vi "MH_T2 Read Acq Q_V2.vi"() -> ()   [LabVIEW 2019]
uses:
  <userlib>/MultiHarp150/T2Lib/MH_T2DeltaQMessage.ctl
  <userlib>/MultiHarp150/T2Lib/MH_T2QMessage.ctl
  <userlib>/MultiHarp150/T2Lib/MH_ResizeBuffer.vi
panel:
  in  "buffbits":i32=16
  out "SpBufSze":i32=1000000
  in  "Dbuffsize":i32=100000
  out "Done":bool
  out "TotalRec":i32
  out "TotalTime":u32
  in  "stop":bool
  out "sortie d'erreur":errorcluster caption="ErrorOut"
  out "RollOver":bool
  out "StBufSze":i32=1000000
  in  "entrée d'erreur":errorcluster caption="ErrorIn"
  in  "WIndowW":i32
  in  "Save Data":bool
  in  "StopCh":u32=2
  in  "StartCh":u32=1
  in  "refnum":refnum<file>
  out "DeltaT":u32[](array[numeric])
  out "nActual":i32[](array[numeric])
  out "En Attente":i32[](array[numeric])
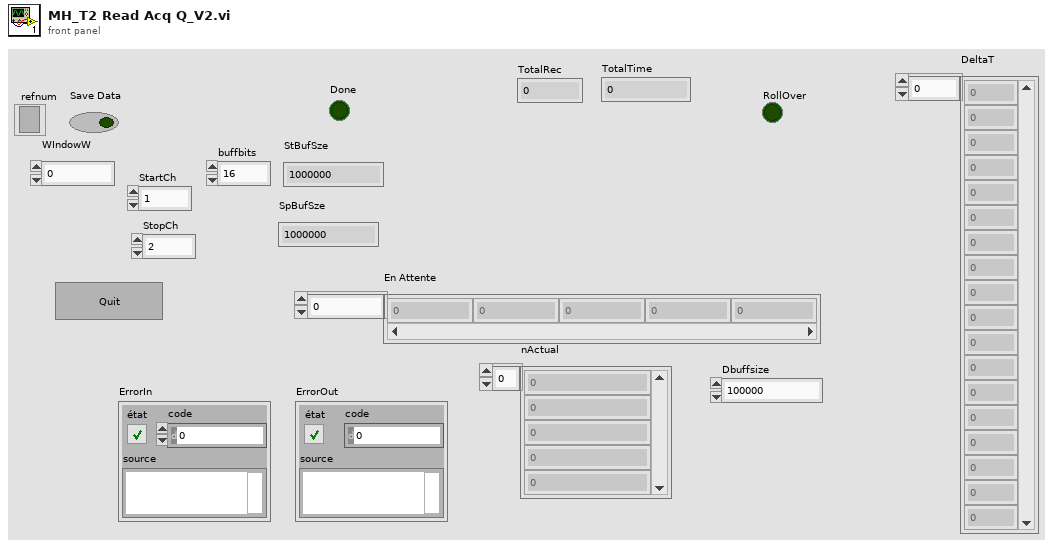
[diagram p1: front panel]
types:
  T1 = typedef "MH_T2DeltaQMessage.ctl" = cluster{"Message":string, "buffer":i32[], "Code":i32, "nactual":i32}
  T2 = typedef "MH_T2QMessage.ctl" = cluster{"Message":string, "buffer":u32[], "Code":i32, "nactual":i32}
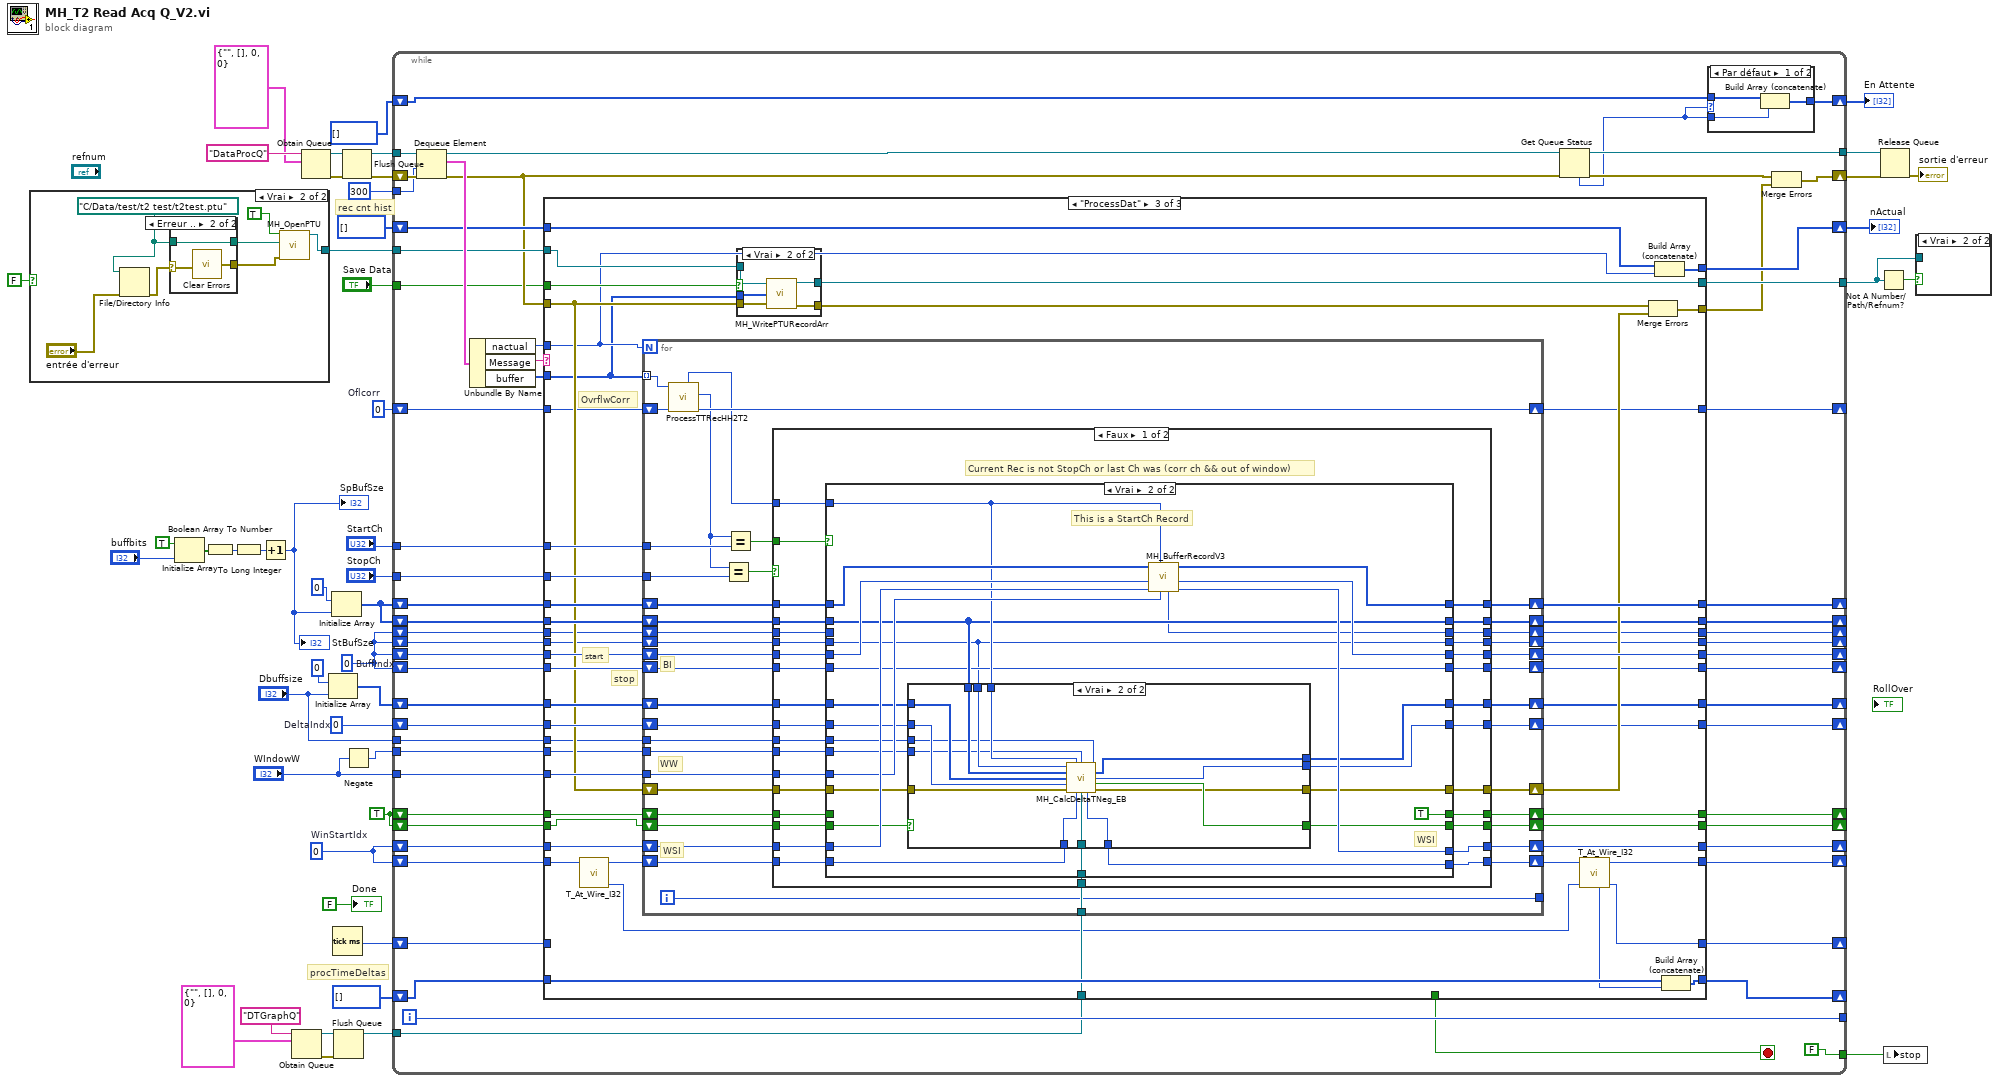
[diagram p0: block diagram]
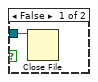
[diagram p2: hidden frame]
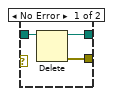
[diagram p4: hidden frame]
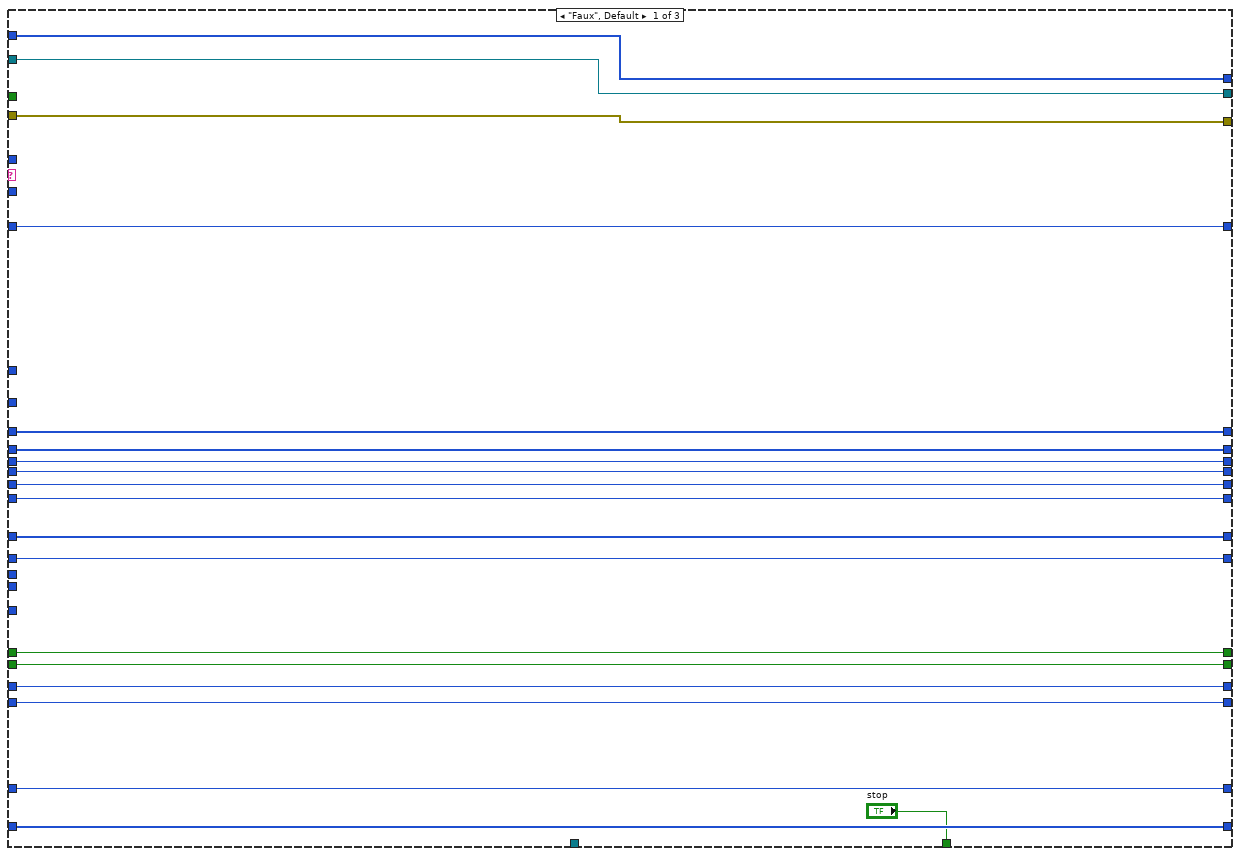
[diagram p6: hidden frame]
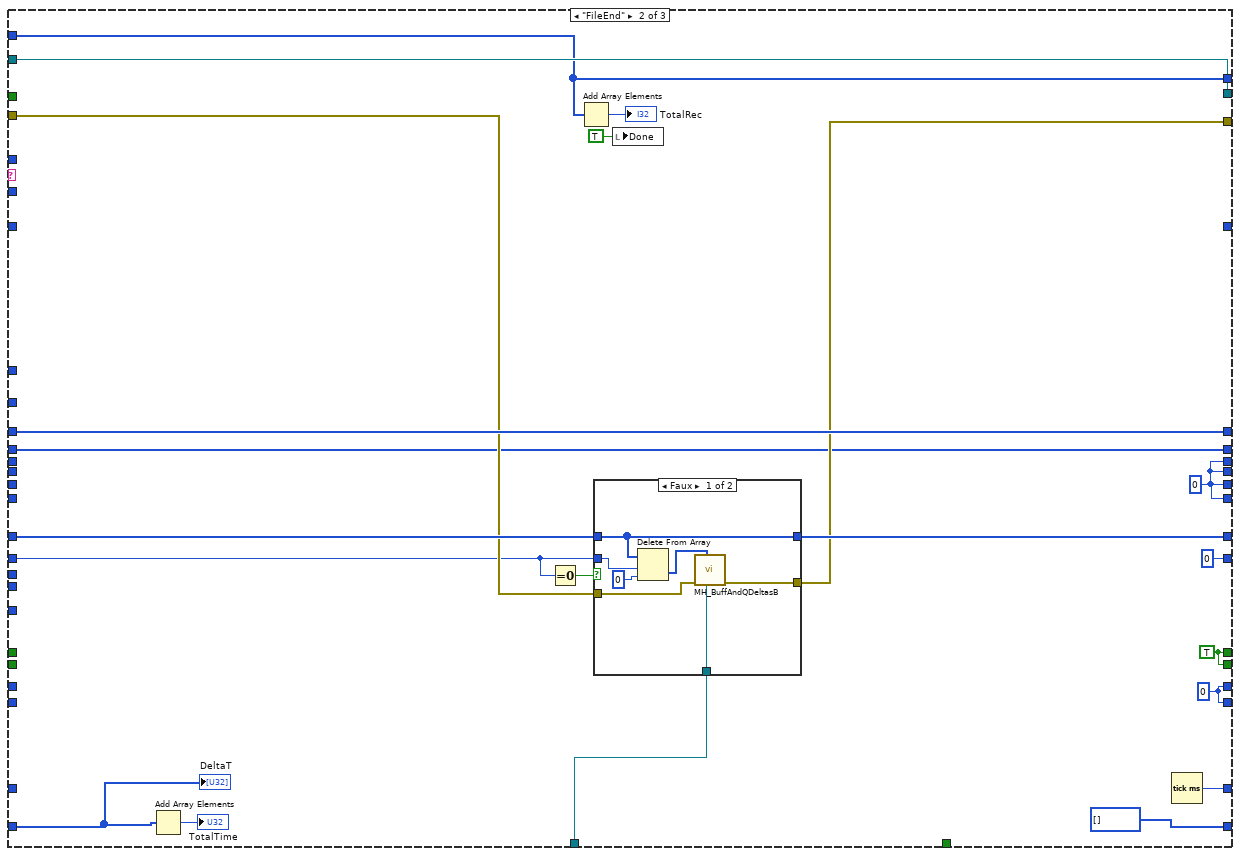
[diagram p7: hidden frame]
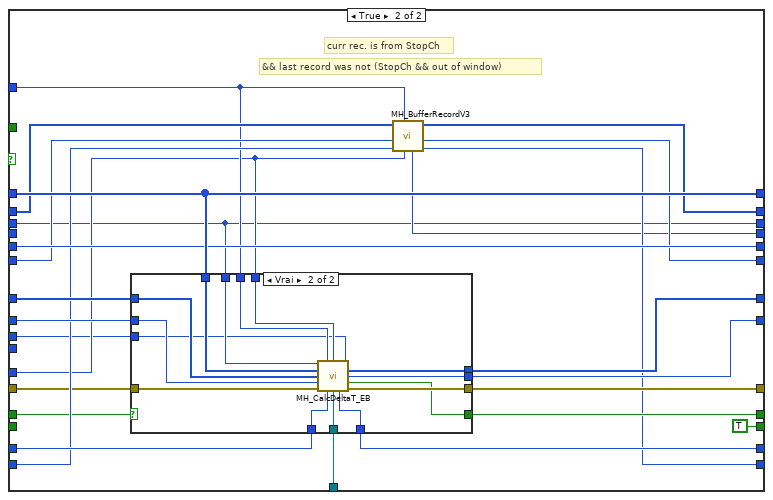
[diagram p12: hidden frame]
diagram:
  w16 = 0  # DeltaIndx
  w12 = TRUE
  w13 = 0  # WinStartIdx
  w1 = 0  # BuffIndx
  w46 = u64 0  # Oflcorr
  # "procTimeDeltas"
  # "rec cnt hist"
  n1 = case shown="Vrai" FALSE {
    tunnel: [_ w54] -> w37
    frame False {
    }
    frame True {
      w51 = path "C:/Data/test/t2 test/t2test.ptu" ("chemin sélectionné")
      n2 = File/Directory Info(path=w51, error in="entrée d'erreur") -> (error out=w50:errorcluster)  [unwired: 6 out]
      n3 = case shown="Erreur .." w50 {
        selector: w50 -> [_ w60]
        tunnel: w51 -> [w58 w61]
        tunnel: [w57 w61] -> w53
        tunnel: [w56 w59] -> w52
        frame No Error {
          n4 = Delete(path (use dialog)=w58) -> (deleted path=w57:path, error out=w56:errorcluster)  [unwired: 4 in, 1 out]
        }
        frame Error {
          n5 = call <vilib>:"Clear Errors.vi"("error in (no error)"=w60) -> ("error out"=w59:errorcluster)  [unwired: 5 in, 1 out]
        }
      }
      n6 = call <userlib>:"MH_OpenPTU.vi"("ErrorIn"=w52, "chemin sélectionné"=w53, "WriteMode"=TRUE) -> ("refnum en sortie"=w54:refnum<file>)  [unwired: 6 in, 2 out]
    }
  }
  n7 = Initialize Array(TRUE, "buffbits") -> (w7:bool[])
  n8 = Boolean Array To Number(Boolean array=w7) -> (number=w5:u32)
  n9 = To Long Integer(number=w5) -> (32bit integer=w3:i32)
  n10 = Increment(x=w3) -> (x+1=w2:i32)
  "StBufSze" <- w2
  "SpBufSze" <- w2
  n11 = Obtain Queue(name (unnamed)="DTGraphQ" ("nom (aucun)"), element data type=T1 {"Message"="", "buffer"=[], "Code"=0, "nactual"=0} ("ClassQueue")) -> (queue out=w18:refnum<queue>, error out=w19:errorcluster)  [unwired: 3 in, 1 out]
  n12 = Obtain Queue(name (unnamed)="DataProcQ" ("nom (aucun)"), element data type=T2 {"Message"="", "buffer"=[], "Code"=0, "nactual"=0} ("ClassQueue")) -> (queue out=w23:refnum<queue>, error out=w20:errorcluster)  [unwired: 3 in, 1 out]
  n13 = Initialize Array(0 ("truetime"), "Dbuffsize") -> (w24:i32[])
  n14 = Initialize Array(u64 0 ("truetime"), w2) -> (w14:u64[])
  n15 = Tick Count (ms)() -> (millisecond timer value=w42:u32)
  n16 = Flush Queue(queue=w18, error in (no error)=w19) -> (queue out=w27:refnum<queue>)  [unwired: 2 out]
  n17 = Flush Queue(queue=w23, error in (no error)=w20) -> (queue out=w22:refnum<queue>, error out=w21:errorcluster)  [unwired: 1 out]
  n18 = Negate(x="WIndowW") -> (-x=w8:i32)
  n19 = while {
    tunnel: w22 -> [w120]
    shift-right: [w100] -> w45
    shift-left: w21 -> [w121]
    shift-right: [w118] -> _
    shift-left: w46 -> [w119]
    tunnel: [w115] -> _
    tunnel: [w111] -> w44
    shift-right: [w109] -> _
    shift-left: w42 -> [w110]
    shift-right: [w107] -> _
    shift-left: u32[] [] ("DeltaT") -> [w108]
    shift-right: [w105] -> w39
    shift-left: i32[] [] ("DeltaT") -> [w106]
    shift-right: [w104] -> w43
    shift-left: i32[] [] ("DeltaT") -> [w103]
    tunnel: w37 -> [w102]
    tunnel: [w99] -> w29
    tunnel: "Save Data" -> [w98]
    shift-right: [w93] -> _
    shift-left: w14 -> [w97]
    shift-right: [w95] -> _
    shift-left: w1 -> [w96]
    tunnel: "StopCh" -> [w94]
    shift-right: [w89] -> _
    shift-left: w13 -> [w92]
    tunnel: "WIndowW" -> [w91]
    tunnel: 300 ("timeout en ms (-1)") -> [w90]
    tunnel: w27 -> [w87]
    shift-right: [w85] -> _
    shift-left: w12 -> [w84]
    shift-right: [w69] -> _
    shift-left: w24 -> [w83]
    tunnel: [FALSE] -> w17
    shift-right: [w78] -> _
    shift-left: w16 -> [w79]
    shift-right: [w72] -> _
    shift-left: w14 -> [w77]
    shift-right: [w73] -> _
    shift-left: w1 -> [w76]
    shift-right: [w74] -> _
    shift-left: w13 -> [w75]
    shift-right: [w70] -> _
    shift-left: w12 -> [w71]
    tunnel: "StartCh" -> [w68]
    tunnel: "Dbuffsize" -> [w67]
    tunnel: w8 -> [w66]
    shift-right: [w65] -> _
    shift-left: w1 -> [w64]
    shift-right: [w63] -> _
    shift-left: w1 -> [w62]
    i -> [w115]
    stop <- w82 stop-if-true
    n20 = Dequeue Element(queue=w120, timeout in ms (-1)=w90, error in (no error)=w121) -> (queue out=w113:refnum<queue>, element=w117:T2, error out=w101:errorcluster)  [unwired: 1 out]
    n21 = Unbundle By Name(w117) -> ("nactual"=w88:i32, "Message"=w114:string, "buffer"=w116:u32[])
    n22 = case shown="\"ProcessDat\"" w114 {
      tunnel: w119 -> [w144 _ w175]
      tunnel: [w144 _ w182] -> w118
      tunnel: w116 -> [_ _ w176]
      tunnel: w110 -> [w143 _ _]
      tunnel: [w142 u32[] [] ("DeltaT") w223] -> w107
      tunnel: [w143 w163 w185] -> w109
      tunnel: w108 -> [w142 w161 w224]
      tunnel: w106 -> [w141 w158 w222]
      tunnel: [w141 w158 w221] -> w105
      tunnel: w102 -> [w128 w165 w197]
      tunnel: w101 -> [w137 w152 w195]
      tunnel: [w128 w165 w192] -> w99
      tunnel: w98 -> [_ _ w196]
      tunnel: w97 -> [w139 w164 w212]
      tunnel: w96 -> [w140 _ w213]
      tunnel: [w140 w145 w219] -> w95
      tunnel: w94 -> [_ _ w220]
      tunnel: [w139 w164 w218] -> w93
      tunnel: w92 -> [w138 _ w207]
      tunnel: w91 -> [_ _ w217]
      tunnel: [w138 w148 w216] -> w89
      tunnel: w88 -> [_ _ w181]
      tunnel: w87 -> [_ w149 w215]
      tunnel: [w137 w153 w194] -> w86
      tunnel: [w136 w146 w211] -> w85
      tunnel: w84 -> [w136 _ w210]
      tunnel: w83 -> [w135 w155 w209]
      tunnel: [w135 w154 w208] -> w69
      tunnel: ["stop" _ _] -> w82
      tunnel: w79 -> [w133 w151 w206]
      tunnel: [w133 0 w205] -> w78
      tunnel: w77 -> [w130 w147 w204]
      tunnel: w76 -> [w131 _ w203]
      tunnel: w75 -> [w132 _ w189]
      tunnel: [w132 w148 w186] -> w74
      tunnel: [w131 w145 w202] -> w73
      tunnel: [w130 w147 w201] -> w72
      tunnel: w71 -> [w129 _ w200]
      tunnel: [w129 w146 w199] -> w70
      tunnel: w68 -> [_ _ w198]
      tunnel: w67 -> [_ _ w191]
      tunnel: w66 -> [_ _ w190]
      tunnel: [w126 w145 w180] -> w65
      tunnel: w64 -> [w126 _ w179]
      tunnel: [w127 w145 w178] -> w63
      tunnel: w62 -> [w127 _ w177]
      frame "Faux", Default {
      }
      frame "FileEnd" {
        w146 = TRUE
        w148 = 0 ("WinStartIdx")
        w145 = 0 ("BuffIndx")
        n23 = Add Array Elements(numeric array=w161) -> (sum=→"TotalTime":u32)
        n24 = Equal To 0?(x=w151) -> (x = 0?=w150:bool)
        n25 = Add Array Elements(numeric array=w158) -> (sum=→"TotalRec":i32)
        n26 = case shown="Faux" w150 {
          tunnel: w155 -> [w169 w174]
          tunnel: [w169 w174] -> w154
          tunnel: [w172 w173] -> w153
          tunnel: w152 -> [w171 w173]
          tunnel: w151 -> [w168 _]
          tunnel: w149 -> [w170 _]
          frame False {
            n27 = Delete From Array(array=w169, length=w168, index=0 ("indice")) -> (deleted portion=w166:i32[])  [unwired: 1 out]
            n28 = call <userlib>:"MH_BuffAndQDeltasB.vi"("queue out"=w170, "DeltasBuffer"=w166, "erroIn"=w171) -> ("error out"=w172:errorcluster)  [unwired: 8 in]
          }
          frame True {
          }
        }
        n29 = local write "Done"(TRUE ("Done")) -> ()
        n30 = Tick Count (ms)() -> (millisecond timer value=w163:u32)
        "DeltaT" <- w161
      }
      frame "ProcessDat" {
        # "stop"
        # "start"
        # "OvrflwCorr"
        n31 = call <userlib>:"T_At_Wire_I32.vi"("I32"=w189) -> ("Clock(ms)"=w183:u32, "I32 Out"=w188:i32)  [unwired: 8 in, 1 out]
        n32 = for {
          N: w181 -> [_]
          tunnel: w176 -> [w232] mode=indexing
          shift-right: [w259] -> w218
          shift-left: w212 -> [w262]
          shift-right: [w260] -> w219
          shift-left: w213 -> [w261]
          tunnel: w220 -> [w270]
          tunnel: w217 -> [w269]
          shift-right: [w268] -> w182
          shift-left: w175 -> [w271]
          shift-right: [w267] -> w216
          shift-left: w207 -> [w264]
          shift-right: [w265] -> w214
          shift-left: w195 -> [w241]
          tunnel: w215 -> [w266]
          shift-right: [w258] -> w211
          shift-left: w210 -> [w257]
          shift-right: [w255] -> w208
          shift-left: w209 -> [w256]
          shift-right: [w253] -> w205
          shift-left: w206 -> [w254]
          tunnel: w198 -> [w252]
          shift-right: [w249] -> w201
          shift-left: w204 -> [w250]
          tunnel: [w251] -> _
          shift-right: [w245] -> w202
          shift-left: w203 -> [w248]
          shift-right: [w246] -> w187
          shift-left: w188 -> [w247]
          shift-right: [w242] -> w199
          shift-left: w200 -> [w243]
          tunnel: w191 -> [w240]
          tunnel: w190 -> [w239]
          shift-right: [w238] -> w180
          shift-left: w179 -> [w237]
          shift-right: [w236] -> w178
          shift-left: w177 -> [w235]
          i -> [w251]
          # "WW"
          # "BI"
          # "WSI"
          n33 = call <userlib>:"ProcessTTRecHH2T2.vi"("oflcorr_in"=w271, "rawbits"=w232) -> ("oflcorr_out"=w268:u64, "channel"=w234:u32, "truetime"=w233:u64)  [unwired: 4 in, 3 out]
          n34 = Equal?(x=w234, y=w270) -> (x = y?=w244:bool)
          n35 = Equal?(x=w234, y=w252) -> (x = y?=w263:bool)
          n36 = case shown="Faux" w244 {
            tunnel: w262 -> [w302 w387]
            tunnel: w264 -> [w298 w385]
            tunnel: w261 -> [w300 w386]
            tunnel: w269 -> [w296 w372]
            tunnel: [w295 w384] -> w267
            tunnel: w266 -> [w282 w365]
            tunnel: [w288 w378] -> w265
            tunnel: w263 -> [w301 _]
            tunnel: w233 -> [w297 w373]
            tunnel: [w299 w386] -> w260
            tunnel: [w303 w387] -> w259
            tunnel: [w294 w381] -> w258
            tunnel: w257 -> [w293 w369]
            tunnel: w256 -> [w278 w383]
            tunnel: [w285 w380] -> w255
            tunnel: w254 -> [w287 w382]
            tunnel: [w286 w379] -> w253
            tunnel: w250 -> [w292 w377]
            tunnel: [w283 w376] -> w249
            tunnel: w248 -> [w291 w375]
            tunnel: w247 -> [w290 w374]
            tunnel: [w289 w371] -> w246
            tunnel: [w284 w370] -> w245
            tunnel: w243 -> [w281 _]
            tunnel: [w280 TRUE ("NewDelta")] -> w242
            tunnel: w241 -> [w279 w367]
            tunnel: w240 -> [w277 w366]
            tunnel: w239 -> [w276 _]
            tunnel: [w275 w363] -> w238
            tunnel: w237 -> [w273 w363]
            tunnel: [w272 w364] -> w236
            tunnel: w235 -> [w274 _]
            frame False {
              # "Current Rec is not StopCh or last Ch was (corr ch && out of window)"
              n37 = case shown="Vrai" w301 {
                tunnel: w302 -> [w315 w336]
                tunnel: w297 -> [_ w331]
                tunnel: w300 -> [w316 w337]
                tunnel: [w316 w341] -> w299
                tunnel: [w315 w340] -> w303
                tunnel: w298 -> [w314 w338]
                tunnel: w296 -> [_ w333]
                tunnel: [w314 w339] -> w295
                tunnel: [w313 TRUE] -> w294
                tunnel: w293 -> [w313 _]
                tunnel: w292 -> [w308 w328]
                tunnel: w291 -> [w309 w327]
                tunnel: w290 -> [w310 w335]
                tunnel: [w310 w334] -> w289
                tunnel: [w306 w332] -> w288
                tunnel: w287 -> [w311 w323]
                tunnel: [w311 w322] -> w286
                tunnel: [w312 w321] -> w285
                tunnel: w278 -> [w312 w330]
                tunnel: [w309 w327] -> w284
                tunnel: [w308 w328] -> w283
                tunnel: w282 -> [_ w329]
                tunnel: w281 -> [w307 w326]
                tunnel: [w307 w325] -> w280
                tunnel: w279 -> [w306 w324]
                tunnel: w277 -> [_ w320]
                tunnel: w276 -> [_ w319]
                tunnel: [w305 w318] -> w275
                tunnel: w274 -> [w304 w317]
                tunnel: w273 -> [w305 _]
                tunnel: [w304 w317] -> w272
                frame False {
                  # "could be sync or non-relevant channel"
                }
                frame True {
                  # "This is a StartCh Record"
                  # "WSI"
                  n38 = case shown="Vrai" w326 {
                    selector: w326 -> [w347 _]
                    tunnel: w328 -> [_ w362]
                    tunnel: w317 -> [_ w361]
                    tunnel: w335 -> [w346 w360]
                    tunnel: [w346 w357] -> w334
                    tunnel: w330 -> [w344 w356]
                    tunnel: w323 -> [w343 w355]
                    tunnel: w324 -> [w345 w354]
                    tunnel: [w347 w358] -> w325
                    tunnel: [w344 w352] -> w321
                    tunnel: [w343 w351] -> w322
                    tunnel: w329 -> [_ w353]
                    tunnel: [w345 w350] -> w332
                    tunnel: w331 -> [_ w359]
                    tunnel: w320 -> [_ w349]
                    tunnel: w319 -> [_ w348]
                    frame False {
                    }
                    frame True {
                      n39 = call <userlib>:"MH_CalcDeltaTNeg_EB.vi"("WinDelta"=w361, "TrueTime"=w359, "WIndowW"=w348, "DBuffSize"=w349, "Data In"=w362, "DeltasBuffer"=w356, "Deltaindex"=w355, "error In"=w354, "WinIndex"=w360, "queue out"=w353) -> ("DeltasBufferOut"=w352:i32[], "DeltaIndexOut"=w351:i32, "NewDelta"=w358:bool, "WinIndexOut"=w357:i32, "Error Out"=w350:errorcluster)  [unwired: 1 in]
                    }
                  }
                  n40 = call <userlib>:"MH_BufferRecordV3.vi"("WindowWidth"=w333, "truetime"=w331, "WinIndex"=w338, "Buffindex"=w337, "Buffer"=w336) -> ("WinIndexOut"=w339:i32, "BuffIndexOut"=w341:i32, "tableau (n rotations)"=w340:u64[], "WindowDelta"=w318:i32)  [unwired: 2 in, 1 out]
                }
              }
            }
            frame True {
              # "&& last record was not (StopCh && out of window)"
              # "curr rec. is from StopCh"
              n41 = case shown="Vrai" w369 {
                selector: w369 -> [w392 _]
                tunnel: w387 -> [_ w407]
                tunnel: w363 -> [_ w406]
                tunnel: w385 -> [w388 w403]
                tunnel: [w388 w404] -> w384
                tunnel: w383 -> [w390 w402]
                tunnel: w382 -> [w389 w401]
                tunnel: w367 -> [w391 w396]
                tunnel: [w392 w393] -> w381
                tunnel: [w390 w395] -> w380
                tunnel: [w389 w394] -> w379
                tunnel: w365 -> [_ w399]
                tunnel: [w391 w398] -> w378
                tunnel: w373 -> [_ w405]
                tunnel: w372 -> [_ w400]
                tunnel: w366 -> [_ w397]
                frame False {
                }
                frame True {
                  n42 = call <userlib>:"MH_CalcDeltaT_EB.vi"("WinDelta"=w406, "TrueTime"=w405, "WIndowW"=w400, "DBuffSize"=w397, "Data In"=w407, "DeltasBuffer"=w402, "Deltaindex"=w401, "error In"=w396, "WinIndex"=w403, "queue out"=w399) -> ("DeltasBufferOut"=w395:i32[], "DeltaIndexOut"=w394:i32, "NewDelta"=w393:bool, "WinIndexOut"=w404:i32, "Error Out"=w398:errorcluster)  [unwired: 1 in]
                }
              }
              n43 = call <userlib>:"MH_BufferRecordV3.vi"("WindowWidth"=w372, "truetime"=w373, "WinIndex"=w374, "Buffindex"=w375, "Buffer"=w377) -> ("WinIndexOut"=w371:i32, "BuffIndexOut"=w370:i32, "tableau (n rotations)"=w376:u64[], "WindowDelta"=w364:i32)  [unwired: 2 in, 1 out]
            }
          }
        }
        n44 = case shown="Vrai" w196 {
          tunnel: w197 -> [w225 w231]
          tunnel: w195 -> [w226 w230]
          tunnel: [w225 w229] -> w192
          tunnel: [w226 w228] -> w193
          tunnel: w176 -> [_ w227]
          frame False {
          }
          frame True {
            n45 = call <userlib>:"MH_WritePTURecordArr.vi"("refnum"=w231, "TTTR Records"=w227, "error in"=w230) -> ("refnum en sortie"=w229:refnum<file>, "error out"=w228:errorcluster)  [unwired: 6 in]
          }
        }
        n46 = call <userlib>:"T_At_Wire_I32.vi"("InitClock(ms)"=w183, "I32"=w187) -> ("Clock(ms)"=w185:u32, "I32 Out"=w186:i32, "Delta(ms)"=w184:u32)  [unwired: 7 in]
        n47 = Merge Errors(w193, w214) -> (w194:errorcluster)
        n48 = Build Array (concatenate)(w222, w181) -> (w221:i32[])
        n49 = Build Array (concatenate)(w224, w184) -> (w223:u32[])
      }
    }
    n50 = Get Queue Status(queue=w113, error in (no error)=w101) -> (queue out=w111:refnum<queue>, error out=w112:errorcluster, # elements in queue=w80:i32)  [unwired: 1 in, 5 out]
    n51 = case shown="Par défaut" w80 {
      tunnel: w80 -> [w124 _]
      tunnel: [w123 w125] -> w104
      tunnel: w103 -> [w122 w125]
      frame Default {
        n52 = Build Array (concatenate)(w122, w124) -> (w123:i32[])
      }
      frame 0 {
      }
    }
    n53 = Merge Errors(w112, w86) -> (w100:errorcluster)
  }
  "En Attente" <- w43
  "nActual" <- w39
  n54 = Not A Number/Path/Refnum?(number/path/refnum=w29) -> (NaN/Path/Refnum?=w28:bool)
  n55 = Release Queue(queue=w44, error in (no error)=w45) -> (error out=→"sortie d'erreur":errorcluster)  [unwired: 1 in, 2 out]
  n56 = local write "stop"(w17) -> ()
  n57 = case shown="Vrai" w28 {
    tunnel: w29 -> [w408 _]
    frame False {
      n58 = Close File(refnum=w408) -> ()  [unwired: 1 in, 2 out]
    }
    frame True {
    }
  }
  "Done" <- FALSE
